vi "Acquire Data.vi"() -> (0 "시간 웨이브폼":waveform(dbl)(graph))   [LabVIEW 2010]
doc: "이 VI는 LabVIEW Core II 교육과정의 연습문제 2-2에 대한 솔루션입니다.\n\n이 VI는 데이터 수집 (DAQ) 보드로부터 데이터를 얻거나 노이즈가 있는 사인 웨이브폼을 생성합니다. 그리고, 주파수 응답을 계산하고 웨이브폼 그래프에 시간 웨이브폼과 함께 디스플레이합니다. 올바른 에러 핸들링을 위해 에러 클러스터와 [단순 에러 핸들러] VI의 사용을 권장합니다."
uses:
  <vilib>/measure/maspectr.llb/FFT Power Spectrum for 1 Chan.vi
  <vilib>/measure/NI_MABase.lvlib
  <vilib>/measure/NI_MAPro.lvlib
panel:
  in  "탭 컨트롤":enum32{"시뮬레이션"}(tab)
  in  "샘플링 정보":cluster{"주파수":dbl, "개수":dbl}={"주파수"=1000.0, "개수"=500.0} {"개수" format="%0.2p"; "주파수" format="%0.2p"}
  in  "노이즈 진폭":dbl(slide)=1.0 scale=0.0..10.0
  in  "사인파 진폭":dbl(slide)=1.0 scale=0.0..10.0
  in  "사인파 주파수":dbl(slide)=100.0 scale=0.0..500.0 scale format="%0.1f"
  in  "평균화 연산 파라미터Parameters":T1={"averaging mode"=enum."No averaging", "weighting mode"=enum."Exponential", "number of averages"=10} caption="평균화 연산 파라미터" {"number of averages" min=1}
  in  "정지":bool
  out "파워 스펙트럼":cluster{"f0":dbl, "df":dbl, "magnitude":dbl[]}(graph)
  # "시뮬레이션 탭의 파라미터를 조절하여 데이터를 변경해 봅니다.  평균화 연산 파라미터의\n선택사항을 변경하여 다르게 데이터를 처리할 수 있습니다.  완료시 계속을 누릅니다."
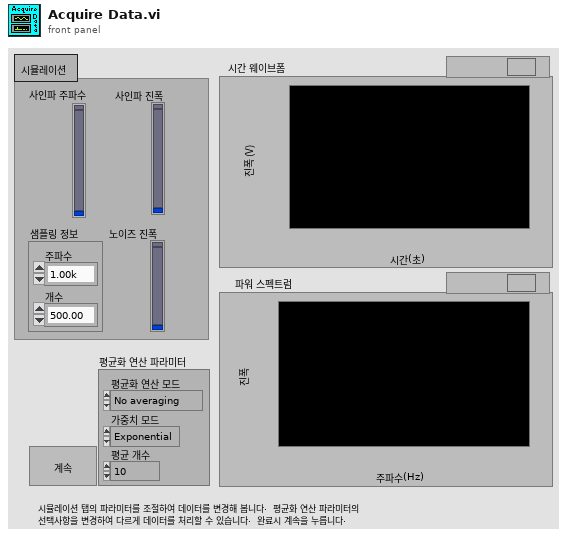
[diagram p1: front panel]
types:
  T1 = cluster{"averaging mode":enum16{"No averaging", "Vector averaging", "RMS averaging", "Peak hold"}, "weighting mode":enum16{"Linear", "Exponential"}, "number of averages":u32}
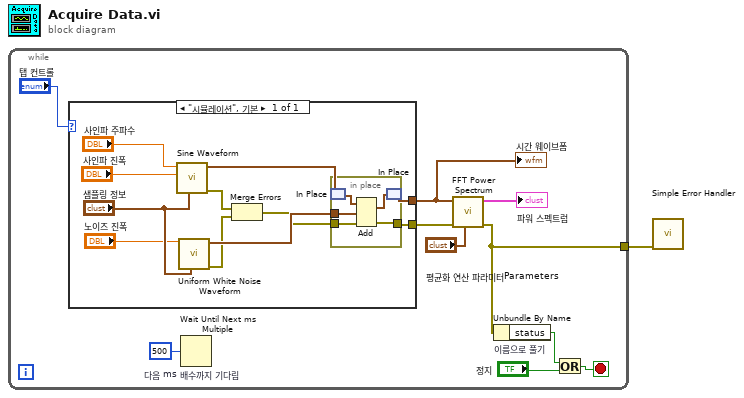
[diagram p0: block diagram]
diagram:
  n1 = while {
    tunnel: [w4] -> w1
    stop <- w5 stop-if-true
    n2 = case shown="\"시뮬레이션\", 기본" "탭 컨트롤" {
      tunnel: [w17] -> w11
      tunnel: [w16] -> w3
      frame "시뮬레이션", Default {
        n3 = call <vilib>:"Sine Waveform.vi"("sampling info"="샘플링 정보", "amplitude"="사인파 진폭", "frequency"="사인파 주파수") -> ("error out"=w19:errorcluster, "signal out"=w22:waveform(dbl))  [unwired: 7 in]
        n4 = call <vilib>:"Uniform White Noise Waveform.vi"("sampling info"="샘플링 정보", "amplitude"="노이즈 진폭") -> ("error out"=w20:errorcluster, "signal out"=w21:waveform(dbl))  [unwired: 8 in]
        n5 = Merge Errors(w19, w20) -> (w18:errorcluster)
        n6 = in-place {
          in-place-border: w21 -> [w26]
          in-place-border: w18 -> [w25]
          in-place-border: [w24] -> w17
          n7 = in-place-match #1(w22) -> (w27:waveform(dbl))
          n8 = Add(1:w26, 2:w27, 4:w25) -> (0:w23:waveform(dbl), 3:w24:errorcluster)
          n9 = in-place-match #1(w23) -> (w16:waveform(dbl))
        }
      }
    }
    "시간 웨이브폼" <- w3
    n10 = Wait Until Next ms Multiple "다음 ms 배수까지 기다림"(millisecond multiple=u32 500) -> ()  [unwired: 1 out]
    n11 = call-poly <vilib>:"FFT Power Spectrum.vi"("averaging parameters"="평균화 연산 파라미터Parameters", "error in (no error)"=w11, "time signal"=w3) -> ("error out"=w4:errorcluster, "power spectrum"=→"파워 스펙트럼":cluster{"f0":dbl, "df":dbl, "magnitude":dbl[]})  [unwired: 5 in, 2 out]
    n12 = Unbundle By Name "이름으로 풀기"(w4) -> ("status"=w7:bool)
    n13 = Or(x=w7, y="정지") -> (x .or. y?=w5:bool)
  }
  n14 = call <vilib>:"Simple Error Handler.vi"("error in (no error)"=w1) -> ()  [unwired: 4 in, 5 out]
